vi "Read Application Ref.vi"(11 "Base Attributes in":refnum<class "Base Attributes.lvclass">) -> (2 "Application Ref":refnum<vi>)   [LabVIEW 2025, in "jettl.lvlib" / "Attributes.lvlib" / "Base Attributes.lvclass"]
uses:
  Base Attributes.lvclass
  Base Attributes.lvclass/Base Attributes.ctl
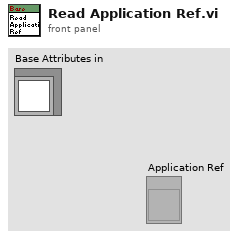
[diagram p1: front panel]
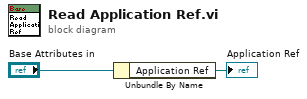
[diagram p0: block diagram]
diagram:
  n1 = Unbundle By Name("Base Attributes in") -> ("Application Ref"=→"Application Ref":refnum<vi>)
